vi "Configured Connection.vi"(8 "error in (no error)":errorcluster, 11 "ConfigPanel in":refnum<class "ConfigPanel.lvclass">) -> (0 "error out":errorcluster, 2 "Configured Connection":refnum<class "Connection.lvclass">, 3 "ConfigPanel out":refnum<class "ConfigPanel.lvclass">)   [LabVIEW 2020, in "LV-Term.lvlib" / "ConfigPanel.lvclass"]
uses:
  ConfigPanel.lvclass
  ConfigPanel.lvclass/ConfigPanel.ctl
  <vilib>/IlluminatedG/lv-stream/Connection/Connection.lvclass
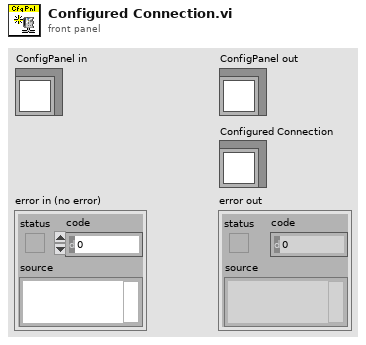
[diagram p1: front panel]
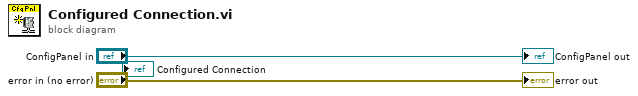
[diagram p0: block diagram]
diagram:
  "error out" <- "error in (no error)"
  "ConfigPanel out" <- "ConfigPanel in"
